vi "Beta 2.2.vi"() -> ()   [LabVIEW 2011]
uses:
  <vilib>/vision/NI_Vision_Development_Module.lvlib
panel:
  in  "Generate":bool
  in  "Look for":enum16{"Bright Objects", "Dark Objects"}(ring)
  in  "Method":T1(ring)=enum."Inter-class Variance"
  out "Binary":T2(plugin-control)
  out "Threshold Range":cluster{"Lower value":sgl, "Upper value":sgl}={"Lower value"=128.0, "Upper value"=255.0} {"Upper value" format="%.2f"; "Lower value" format="%.2f"}
  in  "Stop":bool
  in  "Browse":bool
  out "XY Graph":cluster{dbl[], dbl[]}(graph)
  out "Original Image":T2(plugin-control)
  out "Path to Image":path
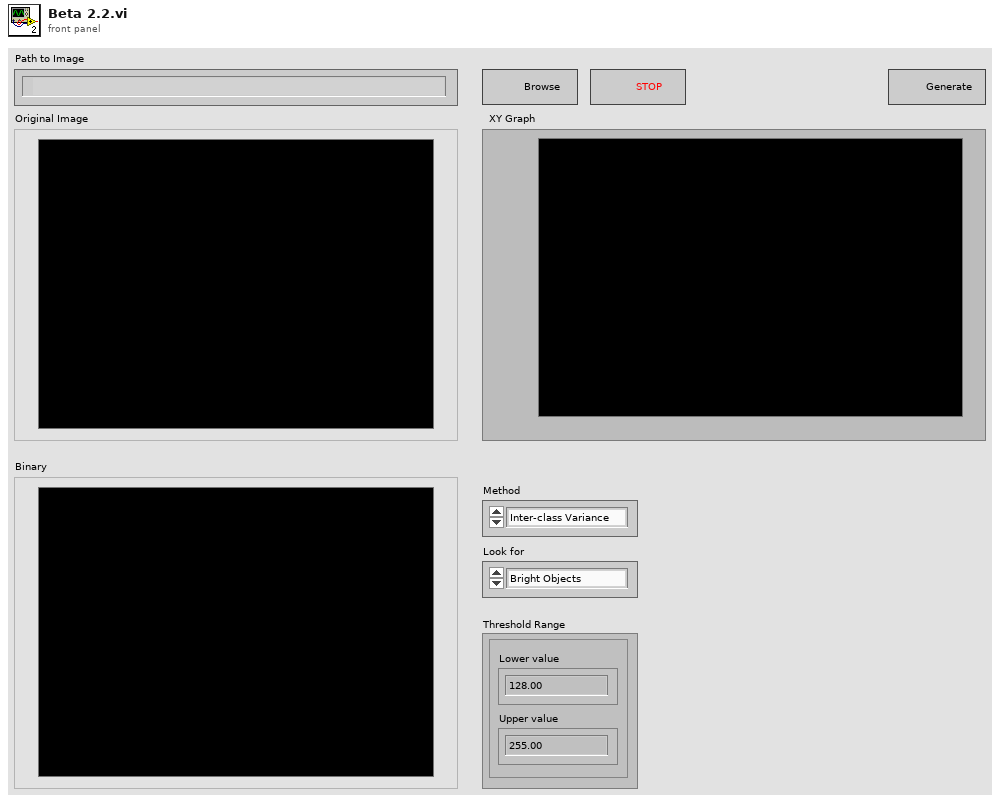
[diagram p1: front panel]
types:
  T1 = enum16{"Clustering", "Entropy", "Metric", "Moments", "Inter-class Variance"}
  T2 = typedef "IMAQ Image.ctl" = refnum<image>
  T3 = typedef "Image Type" = u32
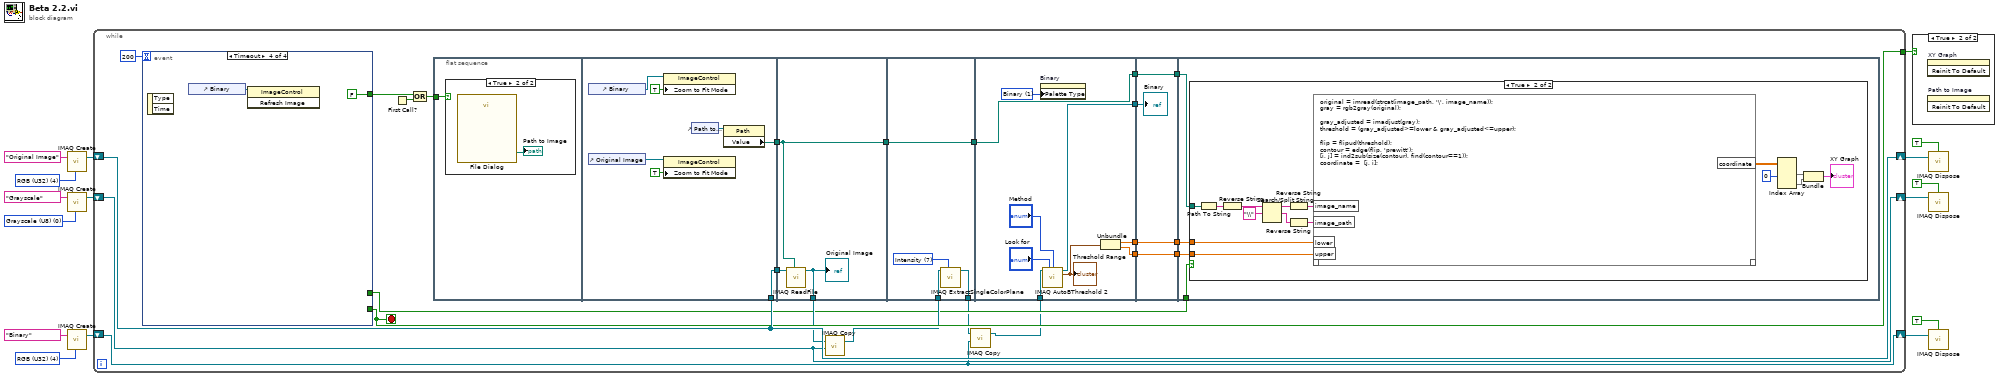
[diagram p0: block diagram]
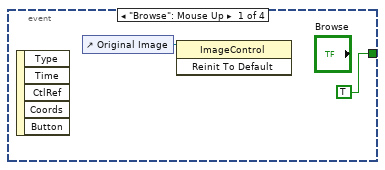
[diagram p3: hidden frame]
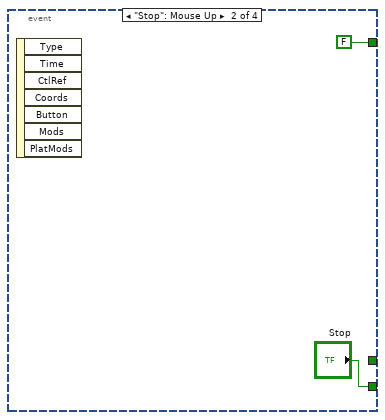
[diagram p4: hidden frame]
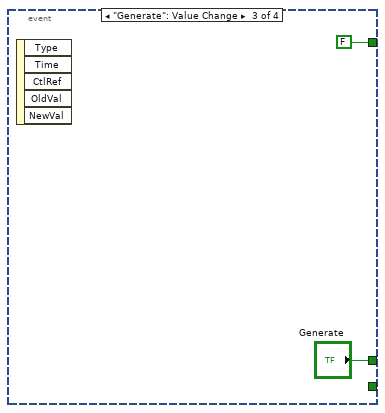
[diagram p5: hidden frame]
diagram:
  w4 = T3 4 items=["Grayscale (U8)", "Grayscale (I16)", "Grayscale (SGL)", "Complex (CSG)", "RGB (U32)", "HSL (U32)", "RGB (U64)", "Grayscale (U16)"] ("Image Type")
  w10 = T3 0 items=["Grayscale (U8)", "Grayscale (I16)", "Grayscale (SGL)", "Complex (CSG)", "RGB (U32)", "HSL (U32)", "RGB (U64)", "Grayscale (U16)"] ("Image Type")
  w15 = T3 4 items=["Grayscale (U8)", "Grayscale (I16)", "Grayscale (SGL)", "Complex (CSG)", "RGB (U32)", "HSL (U32)", "RGB (U64)", "Grayscale (U16)"] ("Image Type")
  n1 = call "IMAQ Create"("Image Name"="Original Image", "Image Type"=w15) -> ("New Image"=w14:T2)  [unwired: 3 in, 1 out]
  n2 = call "IMAQ Create"("Image Name"="Grayscale", "Image Type"=w10) -> ("New Image"=w9:T2)  [unwired: 3 in, 1 out]
  n3 = call "IMAQ Create"("Image Name"="Binary", "Image Type"=w4) -> ("New Image"=w1:T2)  [unwired: 3 in, 1 out]
  n4 = while {
    shift-right: [w35] -> w13
    shift-left: w14 -> [w35]
    tunnel: [w34] -> w12
    shift-right: [w26] -> w7
    shift-left: w9 -> [w26]
    shift-right: [w18] -> w2
    shift-left: w1 -> [w18]
    stop <- w34 stop-if-true
    n5 = event shown="[3] Timeout" {
      selector: _ -> [_ _ _ _]
      dyn-events: _ -> [_ _ _ _]
      timeout: 200 -> [_ _ _ _]
      tunnel: [TRUE FALSE FALSE FALSE] -> w39
      tunnel: [_ "Stop" _ _] -> w34
      tunnel: [_ _ "Generate" _] -> w25
      event "Browse": Mouse Up {
        n6 = event-data() -> ()  [unwired: 1 in, 5 out]
        n7 = control-ref of="Original Image"() -> (w42:refnum<vi>)
        n8 = invoke class="ImageControl" method="Reinit To Default"(reference=w42) -> ()  [unwired: 2 in, 3 out]
      }
      event "Stop": Mouse Up {
        n9 = event-data() -> ()  [unwired: 1 in, 7 out]
      }
      event "Generate": Value Change {
        n10 = event-data() -> ()  [unwired: 1 in, 5 out]
      }
      event Timeout {
        n11 = event-data() -> ()  [unwired: 1 in, 2 out]
        n12 = control-ref of="Binary"() -> (w48:refnum<vi>)
        n13 = invoke class="ImageControl" method="Refresh Image"(reference=w48) -> ()  [unwired: 2 in, 3 out]
      }
    }
    n14 = First Call?() -> (First Call?: T/F=w38:bool)
    n15 = Or(x=w39, y=w38) -> (x .or. y?=w37:bool)
    n16 = flat-sequence {
      tunnel: w37 -> [w49]
      tunnel: [w53] -> w40
      tunnel: [w54] -> w36
      tunnel: w35 -> [w53]
      tunnel: w40 -> [w59]
      tunnel: w36 -> [w60]
      tunnel: [w60] -> w33
      tunnel: [w58] -> w28
      tunnel: w33 -> [w64]
      tunnel: [w64] -> w32
      tunnel: w27 -> [w62]
      tunnel: [w61] -> w19
      tunnel: w32 -> [w73]
      tunnel: [w73] -> w31
      tunnel: [w72] -> w29
      tunnel: [w67] -> w23
      tunnel: [w66] -> w21
      tunnel: w20 -> [w65]
      tunnel: w31 -> [w77]
      tunnel: [w77] -> w30
      tunnel: w29 -> [w76]
      tunnel: [w75] -> w24
      tunnel: w23 -> [w75]
      tunnel: [w74] -> w22
      tunnel: w21 -> [w74]
      tunnel: w30 -> [w81]
      tunnel: w25 -> [w80]
      tunnel: w24 -> [w79]
      tunnel: w22 -> [w78]
      frame #0 {
        n17 = case shown="True" w49 {
          frame False {
          }
          frame True {
            n18 = call "File Dialog"() -> ("selected path"=→"Path to Image":path)  [unwired: 12 in, 3 out]
          }
        }
      }
      frame #1 {
        n19 = control-ref of="Binary"() -> (w52:refnum<vi>)
        n20 = control-ref of="Original Image"() -> (w57:refnum<vi>)
        n21 = property class="ImageControl"(reference=w52, "Zoom to Fit Mode"=TRUE) -> ()  [unwired: 1 in, 2 out]
        n22 = property class="ImageControl"(reference=w57, "Zoom to Fit Mode"=TRUE) -> ()  [unwired: 1 in, 2 out]
        n23 = control-ref of="Path to Image"() -> (w55:refnum<vi>)
        n24 = property class="Path"(reference=w55) -> ("Value"=w54:path)  [unwired: 1 in, 2 out]
      }
      frame #2 {
        n25 = call "IMAQ ReadFile"("File Path"=w60, "Image"=w59) -> ("Image Out"=w58:T2)  [unwired: 5 in, 4 out]
        "Original Image" <- w58
      }
      frame #3 {
        w63 = 7 items=["Red", "Green", "Blue", "Hue", "Saturation", "Luminance", "Value", "Intensity"] ("Color Plane")
        n26 = call "IMAQ ExtractSingleColorPlane"("Color Plane"=w63, "Image Src"=w62) -> ("Image Dst Out"=w61:T2)  [unwired: 8 in, 1 out]
      }
      frame #4 {
        w71 = u32 1 items=["Grayscale", "Binary", "Gradient", "Rainbow", "Temperature", "User Defined"] ("Palette")
        n27 = property on="Binary" class="ImageControl"("Palette Type"=w71) -> ()  [unwired: 2 in, 2 out]
        n28 = call "IMAQ AutoBThreshold 2"("Image Src"=w65, "Look For (Bright Objects)"="Look for", "Method (clustering)"="Method") -> ("Image Dst Out"=w72:T2, "Threshold Range Out"=w68:cluster{"Lower value":sgl, "Upper value":sgl})  [unwired: 10 in, 1 out]
        "Threshold Range" <- w68
        n29 = Unbundle(w68) -> ("Lower value"=w67:sgl, "Upper value"=w66:sgl)
      }
      frame #5 {
        "Binary" <- w76
      }
      frame #6 {
        n30 = case shown="True" w80 {
          tunnel: w81 -> [_ w96]
          tunnel: w79 -> [_ w83]
          tunnel: w78 -> [_ w82]
          frame False {
          }
          frame True {
            n31 = Path To String(path=w96) -> (string=w95:string)
            n32 = Reverse String(1:w95) -> (0:w94:string)
            n33 = Search/Split String(string=w94, search string/char (-)="\\") -> (substring before match=w92:string, match + rest of string=w91:string)  [unwired: 1 in, 1 out]
            n34 = Reverse String(1:w92) -> (0:w90:string)
            n35 = Reverse String(1:w91) -> (0:w89:string)
            n36 = script code="original = imread(strcat(image_path, '\\', image_name));\ngray = rgb2gray(original);\n\ngray_adjusted = imadjust(gray);\nthreshold = (gray_adjusted>=lower & gray_adjusted<=upper);\n\nflip = flipud(threshold);\ncontour = edge(flip, 'prewitt');\n[i, j] = ind2sub(size(contour), find(contour==1));\ncoordinate =  [j, i];"("image_name"=w90, "image_path"=w89, "lower"=w83, "upper"=w82) -> ("coordinate"=w88:dbl[][])  [unwired: 1 in, 1 out]
            n37 = Index Array(array=w88, index (col) #1=0 ("disabled index (col)")) -> (element #1=w87:dbl[], element #2=w86:dbl[])  [unwired: 3 in]
            n38 = Bundle(w87, w86) -> (→"XY Graph":cluster{dbl[], dbl[]})  [unwired: 1 in]
          }
        }
      }
    }
    n39 = call "IMAQ Copy"("Image Dst"=w26, "Image Src"=w28) -> ("Image Dst Out"=w27:T2)  [unwired: 4 in, 1 out]
    n40 = call "IMAQ Copy"("Image Dst"=w18, "Image Src"=w19) -> ("Image Dst Out"=w20:T2)  [unwired: 4 in, 1 out]
  }
  n41 = case shown="True" w12 {
    frame False {
    }
    frame True {
      n42 = invoke on="XY Graph" class="XYGraph (strict)" method="Reinit To Default"() -> ()  [unwired: 3 in, 3 out]
      n43 = invoke on="Path to Image" class="Path" method="Reinit To Default"() -> ()  [unwired: 3 in, 3 out]
    }
  }
  n44 = call "IMAQ Dispose"("All Images? (No)"=TRUE, "Image"=w13) -> ()  [unwired: 4 in, 1 out]
  n45 = call "IMAQ Dispose"("All Images? (No)"=TRUE, "Image"=w7) -> ()  [unwired: 4 in, 1 out]
  n46 = call "IMAQ Dispose"("All Images? (No)"=TRUE, "Image"=w2) -> ()  [unwired: 4 in, 1 out]
